vi "ScanAction.vi"(8 "error in (no error)":errorcluster caption="entrée d'erreur (pas d'erreur)", 9 "IndicePoint":i32, 10 "Dir":bool, 11 "Tools In":refnum<class "Triax320.lvclass"> caption="DNL_LabVIEW Object in") -> (0 "error out":errorcluster caption="sortie d'erreur", 2 "ScanParsOut":dbl[](array[numeric]), 3 "Tools Out":refnum<class "Triax320.lvclass"> caption="DNL_LabVIEW Object out")   [LabVIEW 2019, in "Triax320.lvclass"]
uses:
  Triax320.lvclass
  C:/Programmes Labview/LabScanV1A/DevicesClass/BaseDevice/BaseDevice.lvclass
  Triax320.lvclass/Triax320.ctl
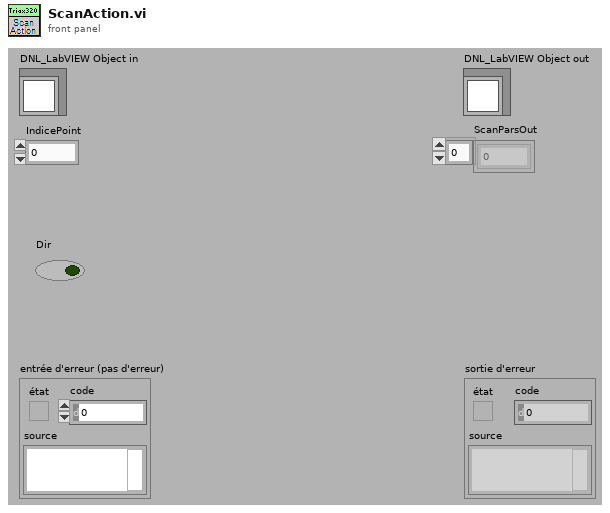
[diagram p1: front panel]
types:
  T1 = typedef "Triax320.lvclass/Triax320_Func.ctl" = enum16{"Position (nm)"}
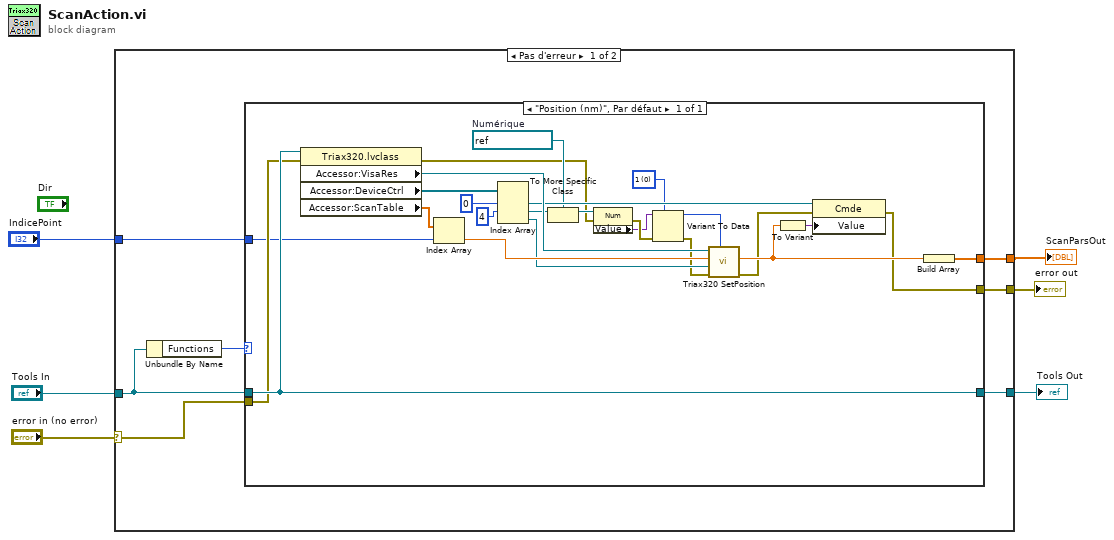
[diagram p0: block diagram]
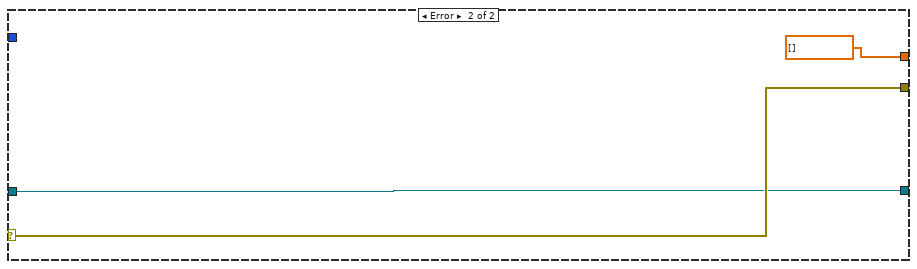
[diagram p2: hidden frame]
diagram:
  n1 = case shown="Pas d'erreur" "error in (no error)" {
    selector: "error in (no error)" -> [w10 w41]
    tunnel: "Tools In" -> [w11 w40]
    tunnel: [w7 dbl[] []] -> w1
    tunnel: [w9 w41] -> w4
    tunnel: [w8 w40] -> w3
    tunnel: "IndicePoint" -> [w12 _]
    frame No Error {
      n2 = Unbundle By Name(w11) -> ("Functions"=w13:T1)
      n3 = case shown="\"Position (nm)\", Par défaut" w13 {
        tunnel: [w38] -> w7
        tunnel: w12 -> [w25]
        tunnel: [w37] -> w8
        tunnel: w11 -> [w37]
        tunnel: w10 -> [w36]
        tunnel: [w28] -> w9
        frame "Position (nm)", Default {
          w16 = u8 0 items=["1", "2", "3"] ("Grating")
          w21 = refnum<vi> refnum  # Numérique
          n4 = property class="Triax320.lvclass"(reference=w37, error in=w36) -> (error out=w19:errorcluster, "Accessor:VisaRes"=w35:refnum<visa-resource-name>, "Accessor:DeviceCtrl"=w27:refnum<vi>[], "Accessor:ScanTable"=w26:dbl[])  [unwired: 1 out]
          n5 = Index Array(array=w26, index=w25) -> (element=w24:dbl)
          n6 = Index Array(array=w27, index #1=0 ("indice"), index #2=4 ("indice")) -> (element #1=w30:refnum<vi>, element #2=w22:refnum<vi>, element #3=w23:refnum<vi>)  [unwired: 1 in]
          n7 = To More Specific Class(target class=w21, reference=w22) -> (specific class reference=w20:refnum<vi>)  [unwired: 1 in, 1 out]
          n8 = property class="Num"(reference=w20, error in=w19) -> (error out=w18:errorcluster, "Value"=w17:variant)  [unwired: 1 out]
          n9 = Variant To Data(error in=w18, type=w16, Variant=w17) -> (data=w15:u8, error out=w14:errorcluster)
          n10 = call <userlib>:"Triax320 SetPosition.vi"("Grating"=w15, "error in (no error)"=w14, "Refnum Cmde"=w23, "Lambda"=w24, "Triax VISA Rsrc"=w35) -> ("error out"=w29:errorcluster, "Lambda Out"=w32:dbl)  [unwired: 3 in, 2 out]
          n11 = To Variant(anything=w32) -> (Variant=w31:variant)
          n12 = property class="Cmde"(reference=w30, error in=w29, "Value"=w31) -> (error out=w28:errorcluster)  [unwired: 1 out]
          n13 = Build Array(w32) -> (w38:dbl[])
        }
      }
    }
    frame Error {
    }
  }
  "error out" <- w4
  "Tools Out" <- w3
  "ScanParsOut" <- w1
